vi "IFA300Configure.vi"(0 "Address":u8, 1 "Port Name":string, 2 "ConfigString":string, 3 "Channel Name":string) -> (8 "Good Echo":bool)   [LabVIEW 2010]
panel:
  out "Array 2":string[](array[string])
  out "Array":bool[](array[boolean])
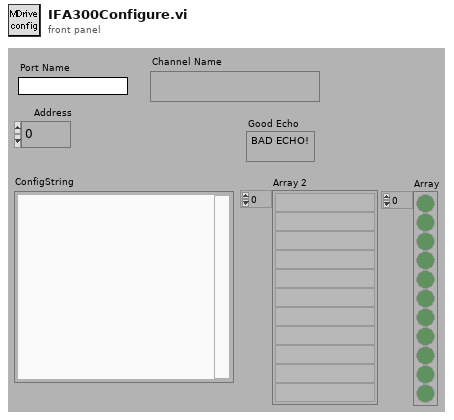
[diagram p1: front panel]
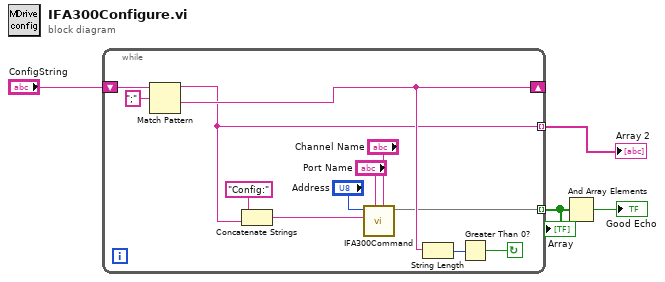
[diagram p0: block diagram]
diagram:
  n1 = while {
    shift-right: [w7] -> _
    shift-left: "ConfigString" -> [w13]
    tunnel: [w6] -> w3 mode=indexing
    tunnel: [w5] -> w1 mode=indexing
    stop <- w9 continue-if-true
    n2 = Match Pattern(string=w13, regular expression=";") -> (before substring=w5:string, after substring=w7:string)  [unwired: 1 in, 2 out]
    n3 = Concatenate Strings("Config:" ("string"), w5) -> (w10:string)
    n4 = call "IFA300Command.vi"("Channel Name"="Channel Name", "Port Name"="Port Name", "IFACommand"=w10, "Address"="Address") -> (3:w6)  [unwired: 3 in, 3 out]
    n5 = String Length(string=w7) -> (length=w8:i32)
    n6 = Greater Than 0?(x=w8) -> (x > 0?=w9:bool)
  }
  "Array" <- w3
  "Array 2" <- w1
  n7 = And Array Elements(Boolean array=w3) -> (logical AND=→"Good Echo":bool)
